vi "TM_datasocket7.vi"() -> ()   [LabVIEW 2018]
panel:
  out "水平进度条":dbl(slide) scale=0.0..100.0
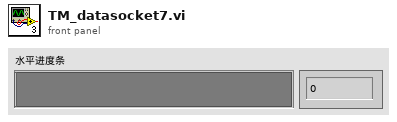
[diagram p1: front panel]
types:
  T1 = enum16{"Read", "Write", "ReadWrite", "BufferedRead", "BufferedReadWrite"}
  T2 = typedef "IMAQ Image.ctl" = refnum<image>
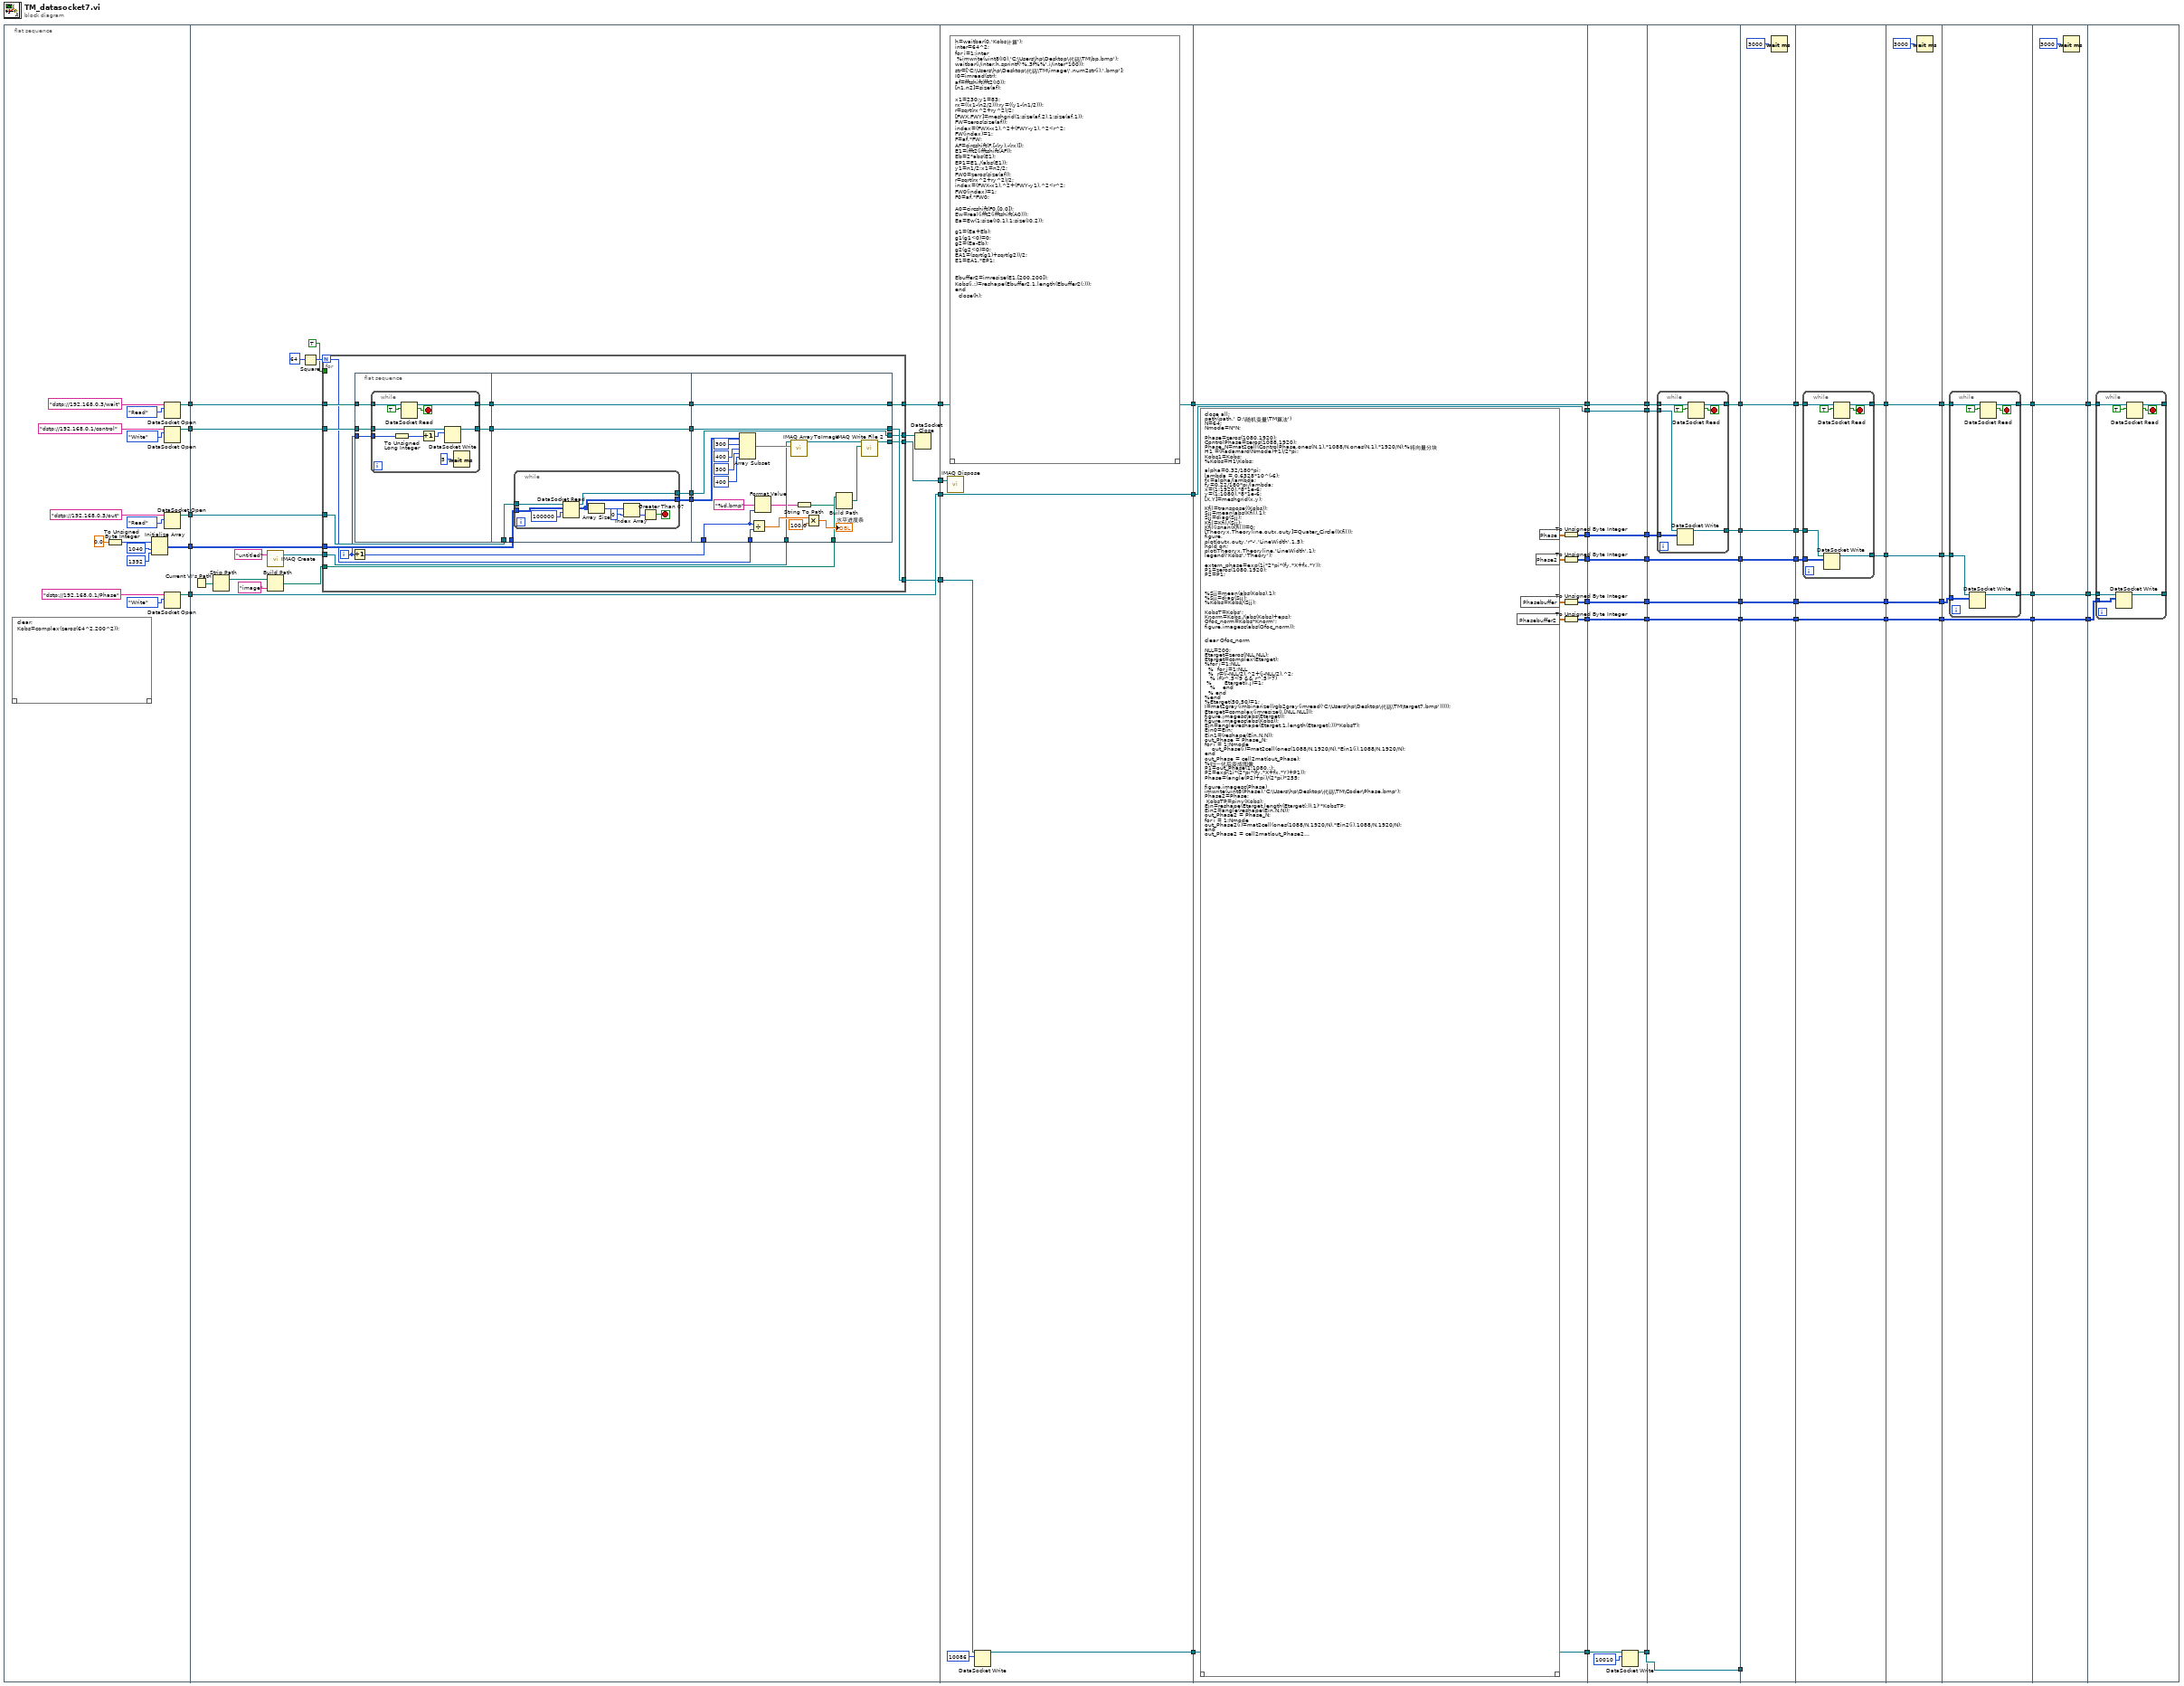
[diagram p0: block diagram]
diagram:
  n1 = flat-sequence {
    tunnel: [w64] -> w51
    tunnel: [w63] -> w50
    tunnel: [w60] -> w49
    tunnel: [w56] -> w48
    tunnel: [w57] -> w47
    tunnel: w51 -> [w84]
    tunnel: w50 -> [w83]
    tunnel: w49 -> [w79]
    tunnel: w48 -> [w82]
    tunnel: [w78] -> w46
    tunnel: w47 -> [w78]
    tunnel: [w77] -> w44
    tunnel: [w76] -> w36
    tunnel: [w69] -> w1
    tunnel: w46 -> [w163]
    tunnel: [w163] -> w45
    tunnel: w44 -> [w162]
    tunnel: [w160] -> w38
    tunnel: [w159] -> w37
    tunnel: w36 -> [w159]
    tunnel: w1 -> [w158]
    tunnel: w45 -> [w174]
    tunnel: [w174] -> w43
    tunnel: [w172] -> w41
    tunnel: [w171] -> w39
    tunnel: w38 -> [w171]
    tunnel: w37 -> [w170]
    tunnel: [w170] -> w34
    tunnel: [w168] -> w27
    tunnel: [w166] -> w20
    tunnel: [w164] -> w2
    tunnel: w43 -> [w183]
    tunnel: [w183] -> w42
    tunnel: w41 -> [w182]
    tunnel: [w182] -> w40
    tunnel: w39 -> [w180]
    tunnel: [w179] -> w35
    tunnel: w34 -> [w179]
    tunnel: [w178] -> w32
    tunnel: w27 -> [w177]
    tunnel: [w177] -> w26
    tunnel: [w176] -> w21
    tunnel: w20 -> [w176]
    tunnel: [w175] -> w3
    tunnel: w2 -> [w175]
    tunnel: w42 -> [w191]
    tunnel: w40 -> [w192]
    tunnel: w35 -> [w190]
    tunnel: [w189] -> w33
    tunnel: w32 -> [w189]
    tunnel: [w188] -> w31
    tunnel: [w187] -> w28
    tunnel: w26 -> [w186]
    tunnel: [w186] -> w25
    tunnel: [w185] -> w22
    tunnel: w21 -> [w185]
    tunnel: [w184] -> w4
    tunnel: w3 -> [w184]
    tunnel: w33 -> [_]
    tunnel: w31 -> [w204]
    tunnel: [w204] -> w30
    tunnel: [w203] -> w29
    tunnel: w28 -> [w203]
    tunnel: w25 -> [w202]
    tunnel: [w202] -> w24
    tunnel: [w201] -> w23
    tunnel: w22 -> [w201]
    tunnel: [w200] -> w5
    tunnel: w4 -> [w200]
    tunnel: w30 -> [w212]
    tunnel: w29 -> [w211]
    tunnel: w24 -> [w210]
    tunnel: w23 -> [w209]
    tunnel: [w209] -> w19
    tunnel: [w208] -> w17
    tunnel: [w207] -> w15
    tunnel: [w206] -> w6
    tunnel: w5 -> [w206]
    tunnel: w19 -> [w224]
    tunnel: [w224] -> w18
    tunnel: w17 -> [w222]
    tunnel: [w222] -> w16
    tunnel: w15 -> [w221]
    tunnel: [w221] -> w14
    tunnel: [w220] -> w7
    tunnel: w6 -> [w220]
    tunnel: w18 -> [w230]
    tunnel: w16 -> [w229]
    tunnel: w14 -> [w228]
    tunnel: [w227] -> w13
    tunnel: [w226] -> w11
    tunnel: [w225] -> w8
    tunnel: w7 -> [w225]
    tunnel: w13 -> [w240]
    tunnel: [w240] -> w12
    tunnel: w11 -> [w239]
    tunnel: [w239] -> w10
    tunnel: [w238] -> w9
    tunnel: w8 -> [w238]
    tunnel: w12 -> [w244]
    tunnel: w10 -> [w243]
    tunnel: w9 -> [w242]
    frame #0 {
      n2 = script code="clear;\nKobs=complex(zeros(64^2,200^2));"() -> ()  [unwired: 1 in, 1 out]
      n3 = To Unsigned Byte Integer(number=0.0 ("元素")) -> (unsigned 8bit integer=w52:u8)
      n4 = Initialize Array(w52, 1040 ("维数大小"), 1392 ("维数大小")) -> (w56:u8[][])
      n5 = DataSocket Open(10:T1."Read" ("模式"), 11:"dstp://192.168.0.3/wait" ("URL")) -> (3:w60:refnum<k13>)  [unwired: 2 in, 1 out]
      n6 = DataSocket Open(10:T1."Write" ("模式"), 11:"dstp://192.168.0.1/control" ("URL")) -> (3:w64:refnum<k13>)  [unwired: 2 in, 1 out]
      n7 = DataSocket Open(10:T1."Read" ("模式"), 11:"dstp://192.168.0.3/out" ("URL")) -> (3:w63:refnum<k13>)  [unwired: 2 in, 1 out]
      n8 = DataSocket Open(10:T1."Write" ("模式"), 11:"dstp://192.168.0.1/Phase" ("URL")) -> (3:w57:refnum<k13>)  [unwired: 2 in, 1 out]
    }
    frame #1 {
      n9 = Current VI's Path() -> (path=w73:path)
      n10 = Strip Path(path=w73) -> (stripped path=w72:path)  [unwired: 1 out]
      n11 = call "IMAQ Create"("Image Name"="untitled") -> ("New Image"=w74:T2)  [unwired: 4 in, 1 out]
      n12 = Build Path(base path=w72, name or relative path="image" ("名称或相对路径")) -> (appended path=w70:path)
      n13 = Square(x=64) -> (x^2=w85:i32)
      n14 = for {
        N: w85 -> [w90]
        tunnel: w84 -> [w92]
        tunnel: [w105] -> w77
        tunnel: w83 -> [w104]
        tunnel: w82 -> [w103]
        tunnel: [w102] -> w81
        tunnel: TRUE -> [_]
        tunnel: w79 -> [w97]
        tunnel: [w94] -> w76
        tunnel: w74 -> [w89]
        tunnel: w70 -> [w88]
        tunnel: [w87] -> w69
        i -> [w93]
        n15 = Increment(x=w93) -> (x+1=w91:i32)
        n16 = flat-sequence {
          tunnel: [w106] -> w98
          tunnel: [w109] -> w95
          tunnel: w93 -> [w108]
          tunnel: w92 -> [w107]
          tunnel: w97 -> [w110]
          tunnel: w98 -> [w126]
          tunnel: w104 -> [w125]
          tunnel: w103 -> [w124]
          tunnel: [w126] -> w101
          tunnel: [w123] -> w100
          tunnel: [w122] -> w99
          tunnel: [w121] -> w96
          tunnel: w95 -> [w121]
          tunnel: [w156] -> w102
          tunnel: [w157] -> w105
          tunnel: w101 -> [w157]
          tunnel: w100 -> [w156]
          tunnel: w99 -> [w150]
          tunnel: w91 -> [w142]
          tunnel: [w155] -> w94
          tunnel: w96 -> [w155]
          tunnel: w90 -> [w154]
          tunnel: w89 -> [w144]
          tunnel: w88 -> [w139]
          tunnel: [w136] -> w87
          frame #0 {
            n17 = while {
              tunnel: w110 -> [w120]
              tunnel: [w117] -> w109
              tunnel: w108 -> [w114]
              tunnel: w107 -> [w113]
              tunnel: [w112] -> w106
              stop <- w118 stop-if-true
              n18 = To Unsigned Long Integer(number=w114) -> (unsigned 32bit integer=w116:u32)
              n19 = DataSocket Read(10:TRUE, 11:w120) -> (2:w118:bool, 3:w117:refnum<k13>)  [unwired: 3 in, 5 out]
              n20 = Increment(x=w116) -> (x+1=w115:u32)
              n21 = DataSocket Write(10:w115, 11:w113) -> (3:w112:refnum<k13>)  [unwired: 2 in, 2 out]
              n22 = Wait (ms)(milliseconds to wait=u32 5 ("等待时间（毫秒）")) -> ()  [unwired: 1 out]
            }
          }
          frame #1 {
            n23 = while {
              tunnel: w125 -> [w135]
              tunnel: [w133] -> w123
              tunnel: w124 -> [w134]
              tunnel: [w131] -> w122
              stop <- w130 stop-if-true
              n24 = DataSocket Read(9:100000 ("毫秒超时(10000)"), 10:w134, 11:w135) -> (2:w131:u8[][], 3:w133:refnum<k13>)  [unwired: 2 in, 5 out]
              n25 = Array Size(array=w131) -> (size(s)=w129:i32[])
              n26 = Index Array(array=w129, index=0 ("索引")) -> (element=w127:i32)
              n27 = Greater Than 0?(x=w127) -> (x > 0?=w130:bool)
            }
          }
          frame #2 {
            n28 = Array Subset(array=w150, index (row)=300 ("索引"), length (row)=400 ("长度"), index (col)=300 ("索引"), length (col)=400 ("长度")) -> (w145:u8[][])
            n29 = Divide(x=w142, y=w154) -> (x/y=w153:dbl)
            n30 = Format Value(format string="%d.bmp" ("格式字符串"), value (0)=w142) -> (output string=w140:string)  [unwired: 1 in]
            n31 = call "IMAQ ArrayToImage"("Image Pixels (U8)"=w145, "Image"=w144) -> ("Image Out"=w143:T2)  [unwired: 8 in, 1 out]
            n32 = String To Path(string=w140) -> (path=w138:path)
            n33 = Multiply(x=w153, y=100.0) -> (x*y=→"水平进度条":dbl)
            n34 = Build Path(base path=w139, name or relative path=w138) -> (appended path=w137:path)
            n35 = call-poly "IMAQ Write File 2"("File Path"=w137, "Image"=w143) -> ("Image Out (duplicate)"=w136:T2)  [unwired: 8 in, 1 out]
          }
        }
      }
      n36 = DataSocket Close(11:w81) -> ()  [unwired: 2 in, 2 out]
    }
    frame #2 {
      n37 = call "IMAQ Dispose"("Image"=w158) -> ()  [unwired: 5 in, 1 out]
      n38 = script code="h=waitbar(0,'Kobs计算');\ninter=64^2;\nfor i=1:inter\n %imwrite(uint8(I0),'C:\\Users\\hp\\Desktop\\代码\\TM\\bp.bmp');\nwaitbar(i/inter,h,sprintf('%.3f%%',i/inter*100));\nstr=['C:\\Users\\hp\\Desktop\\代码\\TM\\image\\',num2str(i),'.bmp'];\nI0=imread(str);\naf=fftshift(fft2(I0));\n[n1,n2]=size(af);\n\nx1=230;y1=83;\nrx=((x1-(n2/2)));ry=((y1-(n1/2)));\nr=sqrt(rx^2+ry^2)/2;\n[FWX,FWY]=meshgrid(1:size(af,2),1:size(af,1));\nFW=zeros(size(af));\nindex=(FWX-x1).^2+(FWY-y1).^2<r^2;\nFW(index)=1;\nF=af.*FW;\nAF=circshift(F,[-(ry),-(rx)]);\nE1=ifft2(ifftshift(AF));\nEb=2*abs(E1);\nEP1=E1./(abs(E1));\ny1=n1/2;x1=n2/2;\nFW0=zeros(size(af));\nr=sqrt(rx^2+ry^2)/2;\nindex=(FWX-x1).^2+(FWY-y1).^2<r^2;\nFW0(index)=1;\nF0=af.*FW0;\n\nA0=circshift(F0,[0,0]);\nEw=real(ifft2(ifftshift(A0)));\nEa=Ew(1:size(I0,1),1:size(I0,2));\n\ng1=(Ea+Eb);\ng1(g1<0)=0;\ng2=(Ea-Eb);\ng2(g2<0)=0;\nEA1=(sqrt(g1)+sqrt(g2))/2;\nE1=EA1.*EP1;\n\n\nEbuffer2=imresize(E1,[200,200]);\nKobs(i,:)=reshape(Ebuffer2,1,length(Ebuffer2(:)));\nend\n  close(h);"() -> ()  [unwired: 1 in, 1 out]
      n39 = DataSocket Write(10:10086, 11:w162) -> (3:w160:refnum<k13>)  [unwired: 2 in, 2 out]
    }
    frame #3 {
      n40 = script code="close all;\npath(path,' D:\\随机变量\\TM算法')\nN=64;\nNmode=N*N;\n\nPhase=zeros(1080,1920);\nControlPhase=zeros(1088,1920);\nPhase_N=mat2cell(ControlPhase,ones(N,1).*1088/N,ones(N,1).*1920/N);%将向量分块\nH1 =(hadamard(Nmode)+1)/2*pi; \nKobs1=Kobs;\n%Kobs=H1\\Kobs;\n\nalpha=0.32/180*pi;\nlambda = 0.6328*10^(-6);\nfx=alpha/lambda;\nfy=0.22/180*pi/lambda;\nx=(1:1920).*8*1e-6;\ny=(1:1080).*8*1e-6;\n[X,Y]=meshgrid(x,y);\n\nKfil=transpose((Kobs));\nSjj=mean(abs(Kfil),1); \nSjj=diag(Sjj);\nKfil=Kfil/(Sjj);\nKfil(isnan(Kfil))=0;\n[Theoryx,Theoryline,outx,outy]=Quater_Circle((Kfil));\nfigure,\nplot(outx,outy,'r*-','LineWidth',1.5);\nhold on;\nplot(Theoryx,Theoryline,'LineWidth',1);\nlegend('Kobs','Theory');\n\nextern_phase=exp(1i*2*pi*(fy.*X+fx.*Y));\nP1=zeros(1080,1920);\nP2=P1;\n\n\n\n%Sjj=mean(abs(Kobs),1);\n%Sjj=diag(Sjj);\n%Kobs=Kobs/(Sjj);\n\nKobsT=Kobs';\nKnorm=Kobs./(abs(Kobs)+eps);\nOfoc_norm=Kobs*Knorm';\nfigure,imagesc(abs(Ofoc_norm));\n\n\nclear Ofoc_norm\n\nNLL=200;\nEtarget=zeros(NLL,NLL);\nEtarget=complex(Etarget);\n%for i=1:NLL\n  %  for j=1:NLL\n  %  r=(i-NLL/2).^2+(j-NLL/2).^2;\n   % if(r^.5<9 && r^.5>7)\n %       Etarget(i,j)=1;\n   %    end\n  % end\n%end\n%Etarget(50,50)=1;\nI=mat2gray(imbinarize((rgb2gray(imread('C:\\Users\\hp\\Desktop\\代码\\TM\\target7.bmp')))));\nEtarget=complex(imresize(I,[NLL,NLL]));\nfigure,imagesc(abs(Etarget));\nfigure,imagesc(abs(Kobs));\nEin=angle(reshape(Etarget,1,length(Etarget(:)))*KobsT);\nEin0=Ein;\nEin1=(reshape(Ein,N,N));\nout_Phase = Phase_N;\nfor i = 1:Nmode\n    out_Phase(i)=mat2cell(ones(1088/N,1920/N).*Ein1(i),1088/N,1920/N);\nend\nout_Phase = cell2mat(out_Phase);\n%归一化后变成图像\nP1=out_Phase(1:1080,:);\nP2=exp(1i*(2*pi*(fy.*X+fx.*Y)+P1));\nPhase=(angle(P2)+pi)/(2*pi)*255;\n\nfigure,imagesc(Phase)\nimwrite(uint8(Phase),'C:\\Users\\hp\\Desktop\\代码\\TM\\Coder\\Phase.bmp');\nPhase2=Phase;\n KobsTP=pinv(Kobs);\nEin=reshape(Etarget,length(Etarget(:)),1)'*KobsTP;\nEin2=angle(reshape(Ein,N,N));\nout_Phase2 = Phase_N;\nfor i = 1:Nmode\nout_Phase2(i)=mat2cell(ones(1088/N,1920/N).*Ein2(i),1088/N,1920/N);\nend\nout_Phase2 = cell2mat(out_Phase2);\nP1=out_Phase2(1:1080,:);\nP2=exp(1i*(2*pi*(fy.*X+fx.*Y)+P1));\nPhase2=(angle(P2)+pi)/(2*pi)*255;\n\nfigure,imagesc(Phase2)\nimwrite(uint8(Phase2),'C:\\Users\\hp\\Desktop\\代码\\TM\\Coder\\Phase2.bmp');\n\ninter=1000;\nU0=ones(size(Phase2)).*exp(1i*Phase2);\nPhasebuffer=Phase2;\nUinverse_phase=angle(Ein)+pi;\nEtarget1=reshape(Etarget,length(Etarget(:)),1);\nfor k=1:inter\n \n    Uout=(ones(length(Uinverse_phase),1)'*255.*exp(1i*Uinverse_phase))*Kobs;\n    Uinverse_in=exp(1i*angle(Uout)).*abs(Etarget1)';\n    Uinverse_out=Uinverse_in*KobsTP;\n    Uinverse_phase=angle(Uinverse_out);\n\nend\nUout=reshape(Uout,NLL,NLL);\nfigure,imagesc(abs(Uout));\nout_Phasebuffer = Phase_N;\n    for i = 1:Nmode\n      out_Phasebuffer(i)=mat2cell(ones(1088/N,1920/N).*Uinverse_phase(i),1088/N,1920/N);\n    end\nout_Phasebuffer = cell2mat(out_Phasebuffer);\nP1=out_Phasebuffer(1:1080,:);\nP2=exp(1i*(2*pi*(fy.*X+fx.*Y)+P1));\nPhasebuffer=(angle(P2)+pi)/(2*pi)*255;\n\n\nfigure,imagesc(Phasebuffer)\nimwrite(uint8(Phasebuffer),'C:\\Users\\hp\\Desktop\\代码\\TM\\Coder\\Phasebuffer2000.bmp');\n\n\nAout=Y_G_Algorithm(Kobs,Etarget1,angle(Ein)+pi,inter);\nout_Phasebuffer2= Phase_N;\nfor i = 1:Nmode\n      out_Phasebuffer2(i)=mat2cell(ones(1088/N,1920/N).*Aout(i),1088/N,1920/N);\n end\nout_Phasebuffer2 = cell2mat(out_Phasebuffer2);\nP1=out_Phasebuffer2(1:1080,:);\nP2=exp(1i*(2*pi*(fy.*X+fx.*Y)+P1));\nPhasebuffer2=(angle(P2)+pi)/(2*pi)*255;\n\nimwrite(uint8(Phasebuffer2),'C:\\Users\\hp\\Desktop\\代码\\TM\\Coder\\Phasebuffer22000.bmp');\n\n\nBout=GA_P(Kobs,Etarget1,inter,64);\nout_Phasebuffer3= Phase_N;\nfor i = 1:Nmode\n      out_Phasebuffer2(i)=mat2cell(ones(1088/N,1920/N).*Bout(i),1088/N,1920/N);\n end\nout_Phasebuffer3= cell2mat(out_Phasebuffer2);\nP1=out_Phasebuffer3(1:1080,:);\nP2=exp(1i*(2*pi*(fy.*X+fx.*Y)+P1));\nPhasebuffer3=(angle(P2)+pi)/(2*pi)*255;\nimwrite(uint8(Phasebuffer3),'C:\\Users\\hp\\Desktop\\代码\\TM\\Coder\\Phasebuffer32000.bmp');"() -> ("Phase"=w173:dbl[][], "Phase2"=w169:dbl[][], "Phasebuffer"=w167:dbl[][], "Phasebuffer2"=w165:dbl[][])  [unwired: 1 in, 1 out]
      n41 = To Unsigned Byte Integer(number=w173) -> (unsigned 8bit integer=w172:u8[][])
      n42 = To Unsigned Byte Integer(number=w169) -> (unsigned 8bit integer=w168:u8[][])
      n43 = To Unsigned Byte Integer(number=w167) -> (unsigned 8bit integer=w166:u8[][])
      n44 = To Unsigned Byte Integer(number=w165) -> (unsigned 8bit integer=w164:u8[][])
    }
    frame #4 {
      n45 = DataSocket Write(10:10010, 11:w180) -> (3:w178:refnum<k13>)  [unwired: 2 in, 2 out]
    }
    frame #5 {
      n46 = while {
        tunnel: w192 -> [w199]
        tunnel: w190 -> [w196]
        tunnel: [w193] -> w187
        tunnel: w191 -> [w197]
        tunnel: [w198] -> w188
        stop <- w194 stop-if-true
        n47 = DataSocket Write(10:w199, 11:w197) -> (3:w198:refnum<k13>)  [unwired: 2 in, 2 out]
        n48 = DataSocket Read(10:TRUE, 11:w196) -> (2:w194:bool, 3:w193:refnum<k13>)  [unwired: 3 in, 5 out]
      }
    }
    frame #6 {
      n49 = Wait (ms)(milliseconds to wait=u32 3000 ("等待时间（毫秒）")) -> ()  [unwired: 1 out]
    }
    frame #7 {
      n50 = while {
        tunnel: w210 -> [w219]
        tunnel: w211 -> [w216]
        tunnel: [w213] -> w207
        tunnel: w212 -> [w217]
        tunnel: [w218] -> w208
        stop <- w214 stop-if-true
        n51 = DataSocket Write(10:w219, 11:w217) -> (3:w218:refnum<k13>)  [unwired: 2 in, 2 out]
        n52 = DataSocket Read(10:TRUE, 11:w216) -> (2:w214:bool, 3:w213:refnum<k13>)  [unwired: 3 in, 5 out]
      }
    }
    frame #8 {
      n53 = Wait (ms)(milliseconds to wait=u32 3000 ("等待时间（毫秒）")) -> ()  [unwired: 1 out]
    }
    frame #9 {
      n54 = while {
        tunnel: w230 -> [w237]
        tunnel: w228 -> [w234]
        tunnel: [w231] -> w226
        tunnel: w229 -> [w235]
        tunnel: [w236] -> w227
        stop <- w232 stop-if-true
        n55 = DataSocket Write(10:w237, 11:w235) -> (3:w236:refnum<k13>)  [unwired: 2 in, 2 out]
        n56 = DataSocket Read(10:TRUE, 11:w234) -> (2:w232:bool, 3:w231:refnum<k13>)  [unwired: 3 in, 5 out]
      }
    }
    frame #10 {
      n57 = Wait (ms)(milliseconds to wait=u32 3000 ("等待时间（毫秒）")) -> ()  [unwired: 1 out]
    }
    frame #11 {
      n58 = while {
        tunnel: w242 -> [w251]
        tunnel: w243 -> [w248]
        tunnel: [w245] -> _
        tunnel: w244 -> [w249]
        tunnel: [w250] -> _
        stop <- w246 stop-if-true
        n59 = DataSocket Write(10:w251, 11:w249) -> (3:w250:refnum<k13>)  [unwired: 2 in, 2 out]
        n60 = DataSocket Read(10:TRUE, 11:w248) -> (2:w246:bool, 3:w245:refnum<k13>)  [unwired: 3 in, 5 out]
      }
    }
  }
